vi "题目8.vi"() -> ()   [LabVIEW 2017]
panel:
  in  "n":dbl
  in  "m":dbl
  in  "x":dbl
  out "y":dbl
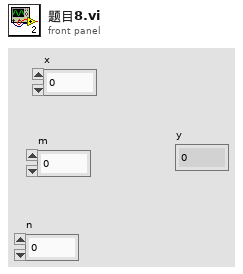
[diagram p1: front panel]
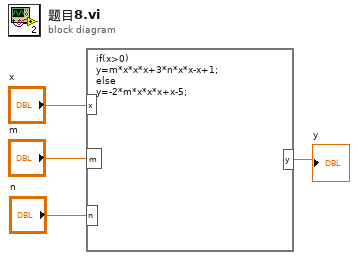
[diagram p0: block diagram]
diagram:
  n1 = formula code="if(x>0)\ny=m*x*x*x+3*n*x*x-x+1;\nelse \ny=-2*m*x*x*x+x-5;"("m"="m", "n"="n", "x"="x") -> ("y"=→"y":dbl)
